vi "Attenuator Unpack and Check Stimulus.vi"(3 "Flat Stimulus":string, 5 "Requested Stimulus In":T1={"ATT Stimulus"={"Normalize"=TRUE, "Value (dB)"=0.0}, "VNA Stimulus"={"Use Instrument Settings"=FALSE, "Blank Frequencies"=FALSE, "Sweep Type"=enum."Linear", "Sweep"={"Fstart"=500.0, "Fstop"=1500.0, "Units"=enum."MHz", "Points"=201}, "Power (dBm)"=999.0, "IFBW (Hz)"=-1.0, "Sweep Time (s)"=-1.0, "Calibration"={"State"=FALSE, "String"=""}}} {"VNA Stimulus"."Sweep Time (s)" format="%.3g"}) -> (0 "Stimulus Changed?":bool, 1 "Current Stimulus":T1={"ATT Stimulus"={"Normalize"=TRUE, "Value (dB)"=0.0}, "VNA Stimulus"={"Use Instrument Settings"=FALSE, "Blank Frequencies"=FALSE, "Sweep Type"=enum."Linear", "Sweep"={"Fstart"=500.0, "Fstop"=1500.0, "Units"=enum."MHz", "Points"=201}, "Power (dBm)"=999.0, "IFBW (Hz)"=-1.0, "Sweep Time (s)"=-1.0, "Calibration"={"State"=FALSE, "String"=""}}} {"VNA Stimulus"."Sweep Time (s)" format="%.3g"}, 2 "Requested Stimulus Out":T1={"ATT Stimulus"={"Normalize"=TRUE, "Value (dB)"=0.0}, "VNA Stimulus"={"Use Instrument Settings"=FALSE, "Blank Frequencies"=FALSE, "Sweep Type"=enum."Linear", "Sweep"={"Fstart"=500.0, "Fstop"=1500.0, "Units"=enum."MHz", "Points"=201}, "Power (dBm)"=999.0, "IFBW (Hz)"=-1.0, "Sweep Time (s)"=-1.0, "Calibration"={"State"=FALSE, "String"=""}}} {"VNA Stimulus"."Sweep Time (s)" format="%.3g"})   [LabVIEW 2011]
uses:
  TypeDefs/Attenuator Stimulus Parameters.ctl
  TypeDefs/Attenuator ATT Stimulus.ctl
  TypeDefs/Attenuator VNA Stimulus.ctl
  S Parameter/TypeDefs/SP Frequency Units.ctl
  TypeDefs/Attenuator VNA Calibration State.ctl
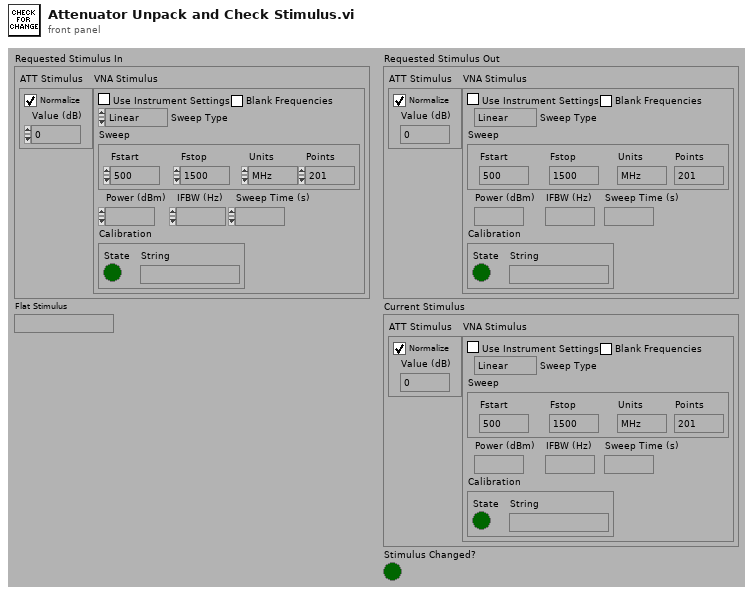
[diagram p1: front panel]
types:
  T1 = typedef "Attenuator Stimulus Parameters.ctl" = cluster{"ATT Stimulus":T2, "VNA Stimulus":T3}
  T2 = typedef "Attenuator ATT Stimulus.ctl" = cluster{"Normalize":bool, "Value (dB)":dbl}
  T3 = typedef "Attenuator VNA Stimulus.ctl" = cluster{"Use Instrument Settings":bool, "Blank Frequencies":bool, "Sweep Type":enum32{"Linear", "Logarithmic", "List", "Power", "CW"}, "Sweep":cluster{"Fstart":dbl, "Fstop":dbl, "Units":T4, "Points":i32}, "Power (dBm)":dbl, "IFBW (Hz)":dbl, "Sweep Time (s)":dbl, "Calibration":T5}
  T4 = typedef "SP Frequency Units.ctl" = enum16{"Hz", "kHz", "MHz", "GHz", "Points"}
  T5 = typedef "Attenuator VNA Calibration State.ctl" = cluster{"State":bool, "String":string}
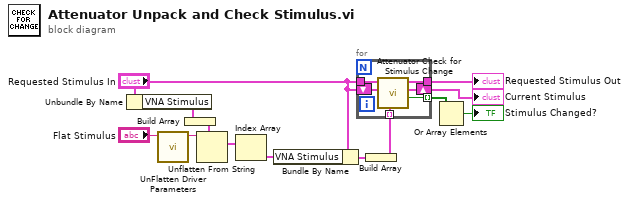
[diagram p0: block diagram]
diagram:
  n1 = Unbundle By Name("Requested Stimulus In") -> ("VNA Stimulus"=w7:T3)
  n2 = call "UnFlatten Driver Parameters.vi"("Flattened Driver Parameters with Version (\"\")"="Flat Stimulus") -> ("Flat Driver Parameters"=w8:string)  [unwired: 1 in, 5 out]
  n3 = Build Array(w7) -> (w6:T3[])
  n4 = Unflatten From String(type=w6, binary string=w8) -> (value=w3:T3[])  [unwired: 1 in, 4 out]
  n5 = Index Array(array=w3) -> (element=w5:T3)  [unwired: 1 in]
  n6 = Bundle By Name(cluster="Requested Stimulus In", "VNA Stimulus"=w5) -> (w4:T1)
  n7 = Build Array(w4) -> (w2:T1[])
  n8 = for {
    tunnel: [w19] -> w9 mode=indexing
    tunnel: [w16] -> w10
    tunnel: w2 -> [w18] mode=indexing
    tunnel: "Requested Stimulus In" -> [w17]
    shift-right: [w14] -> w12
    shift-left: "Requested Stimulus In" -> [w15]
    n9 = call "Attenuator Check for Stimulus Change.vi"("Current Stimulus Channel"=w18, "Current Stimulus In"=w15, "New Stimulus"=w17) -> ("Stimulus Changed?"=w19:bool, "Current Stimulus Out"=w14:T1, "Stimulus to Set"=w16:T1)  [unwired: 6 out]
  }
  "Current Stimulus" <- w12
  "Requested Stimulus Out" <- w10
  n10 = Or Array Elements(Boolean array=w9) -> (logical OR=→"Stimulus Changed?":bool)
